vi "close.vi"(8 "error in":errorcluster, 11 "module in":refnum<class "WaveformAcq runtime.lvclass">) -> (0 "error out":errorcluster)   [LabVIEW 2017, in "WaveformAcq runtime.lvclass"]
doc: "Provides an interface for terminating a module instance. While this interface performs no operations, a child should close and deallocate any open references or memory."
uses:
  WaveformAcq runtime.lvclass
  WaveformAcq runtime.lvclass/WaveformAcq runtime.ctl
  <vilib>/NI/PowerElectronicsControl/WaveformAcq/RT/WaveformTask.lvclass
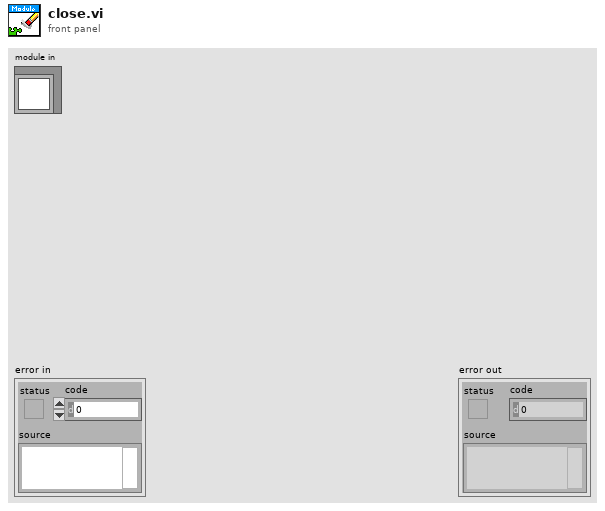
[diagram p1: front panel]
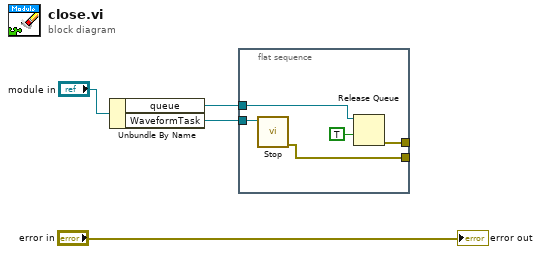
[diagram p0: block diagram]
diagram:
  n1 = Unbundle By Name("module in") -> ("queue"=w2:refnum<queue>, "WaveformTask"=w3:refnum<class "WaveformTask.lvclass">)
  n2 = flat-sequence {
    tunnel: w3 -> [w9]
    tunnel: w2 -> [w8]
    tunnel: [w6] -> _
    tunnel: [w5] -> _
    frame #0 {
      n3 = call <vilib>:"Stop.vi"("WaveformTask in"=w9) -> ("error out"=w5:errorcluster)  [unwired: 9 in, 1 out]
      n4 = Release Queue(queue=w8, force destroy? (F)=TRUE) -> (error out=w6:errorcluster)  [unwired: 1 in, 2 out]
    }
  }
  "error out" <- "error in"
